vi "Resistance Input Example.vi"() -> ()   [LabVIEW 2012, in "Phidget Resistance Input.lvlib"]
uses:
  <instrlib>/Phidgets/Phidget Resistance Input/Phidget Resistance Input.lvlib
  <instrlib>/Phidgets/Phidget Resistance Input/Public/ResistanceInputStart.vi
  <instrlib>/Phidgets/Phidget Resistance Input/Public/ResistanceInputClose.vi
  <instrlib>/Phidgets/Phidget Common/Phidget Common.lvlib
panel:
  out "Resistance":dbl caption="Temperature"
  out "error out":errorcluster
  in  "error in (no error)":errorcluster
  in  "Device Info":T1={"Serial Number"=-1, "Channel"=0, "Port"=0}
  out "Attached?":bool
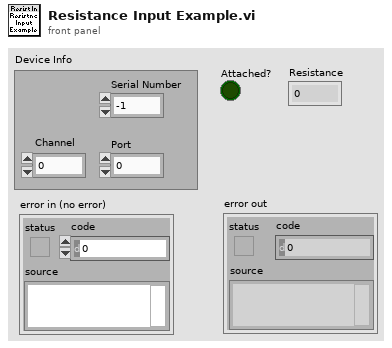
[diagram p1: front panel]
types:
  T1 = cluster{"Serial Number":i32, "Channel":i32, "Port":i32}
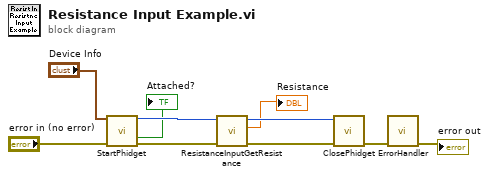
[diagram p0: block diagram]
diagram:
  n1 = call-poly <instrlib>:"StartPhidget.vi"("Device Info"="Device Info", "error in (no error)"="error in (no error)") -> ("Phidget ID"=w10:u64, "Attached?"=→"Attached?":bool, "error out"=w9:errorcluster)  [unwired: 10 in, 1 out]
  n2 = call <instrlib>:"ResistanceInputGetResistance.vi"("error in (no error)"=w9, "Device In"=w10) -> ("error out"=w2:errorcluster, "Resistance"=→"Resistance":dbl, "Device Out"=w3:u64)  [unwired: 6 in]
  n3 = call-poly <instrlib>:"ClosePhidget.vi"("error in"=w2, "Device In"=w3) -> ("error out"=w5:errorcluster)  [unwired: 9 in]
  n4 = call <instrlib>:"ErrorHandler.vi"("error in"=w5) -> ("error out"=→"error out":errorcluster)  [unwired: 9 in, 1 out]
